vi "Display name.vi"(1 "State In":T1) -> (0 "Name":string)   [LabVIEW 2018, in "FilterArray.xnode"]
uses:
  FilterArray.xnode
  State.ctl
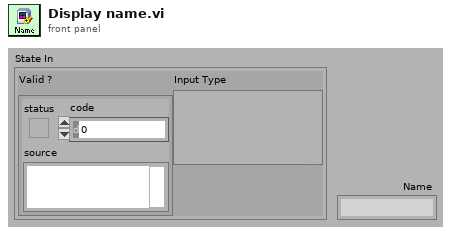
[diagram p1: front panel]
types:
  T1 = typedef "FilterArray.xnode/State.ctl" = cluster{"Valid ?":errorcluster, "Input Type":variant}
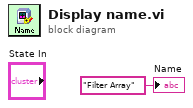
[diagram p0: block diagram]
diagram:
  "Name" <- "Filter Array" ("Name")
